vi "Sub03_01_CheckIfExeExists.vi"(8 "error in (no error)":errorcluster, 11 "vi name":string) -> (0 "error out":errorcluster, 3 "appended path":path)   [LabVIEW 2019]
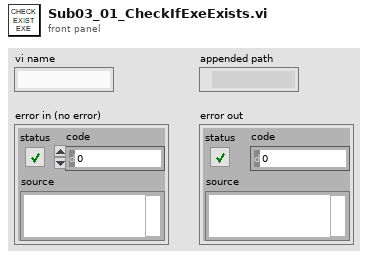
[diagram p1: front panel]
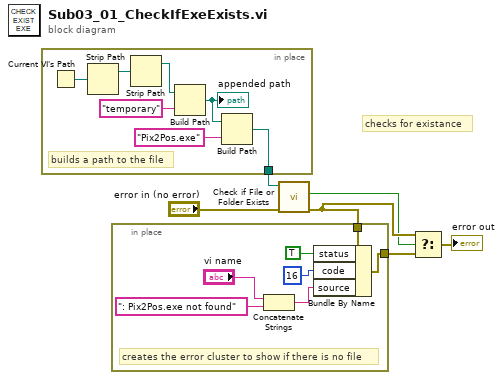
[diagram p0: block diagram]
diagram:
  # "checks for existance"
  n1 = in-place {
    in-place-border: [w8] -> w1
    # "builds a path to the file"
    n2 = Current VI's Path() -> (path=w7:path)
    n3 = Strip Path(path=w7) -> (stripped path=w10:path)  [unwired: 1 out]
    n4 = Strip Path(path=w10) -> (stripped path=w11:path)  [unwired: 1 out]
    n5 = Build Path(base path=w11, name or relative path="temporary") -> (appended path=w12:path)
    "appended path" <- w12
    n6 = Build Path(base path=w12, name or relative path="Pix2Pos.exe") -> (appended path=w8:path)
  }
  n7 = call <vilib>:"Check if File or Folder Exists.vi"("error in (no error)"="error in (no error)", "path"=w1) -> ("error out"=w6:errorcluster, "file or folder exists?"=w2:bool)  [unwired: 7 in, 1 out]
  n8 = in-place {
    in-place-border: w6 -> [w19]
    in-place-border: [w18] -> w5
    # "creates the error cluster to show if there is no file"
    n9 = Concatenate Strings("vi name", ": Pix2Pos.exe not found" ("string")) -> (w17:string)
    n10 = Bundle By Name(cluster=w19, "status"=TRUE, "code"=16, "source"=w17) -> (w18:errorcluster)
  }
  n11 = Select(t=w6, s=w2, f=w5) -> (s? t:f=→"error out":errorcluster)
